vi "WFDC Dynamic Step.vi"(0 "Setpoint":dbl, 2 "Step Size":dbl, 7 "Process Value":dbl, 13 "Gain":dbl) -> (8 "Output":dbl)   [LabVIEW 2016]
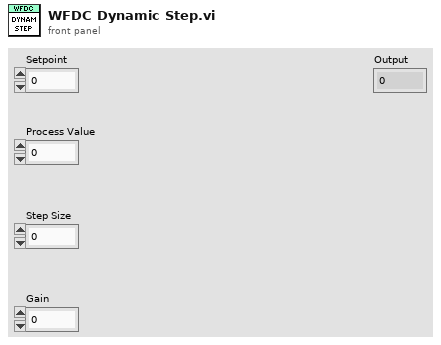
[diagram p1: front panel]
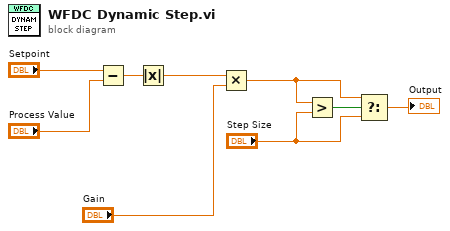
[diagram p0: block diagram]
diagram:
  n1 = Subtract(x="Setpoint", y="Process Value") -> (x-y=w7:dbl)
  n2 = Absolute Value(x=w7) -> (abs(x)=w6:dbl)
  n3 = Multiply(x=w6, y="Gain") -> (x*y=w3:dbl)
  n4 = Greater?(x=w3, y="Step Size") -> (0:w4:bool)
  n5 = Select(t=w3, s=w4, f="Step Size") -> (s? t:f=→"Output":dbl)
